vi "FTW-System-CurrentMemoryStatistics.vi"(11 "error in":errorcluster) -> (4 "DS Bytes Allocated":i64 format="%_4pbytes", 15 "error out":errorcluster)   [LabVIEW 2014]
uses:
  error/FTW-ERR-ThrowGenericError.vi
  error/FTW-ERR-ThrowError.vi
  error/FTW-ERR-CallChain.vi
  string/FTW-STR-ReplaceWhitespace.vi
panel:
  # "Inputs"
  # "Outputs"
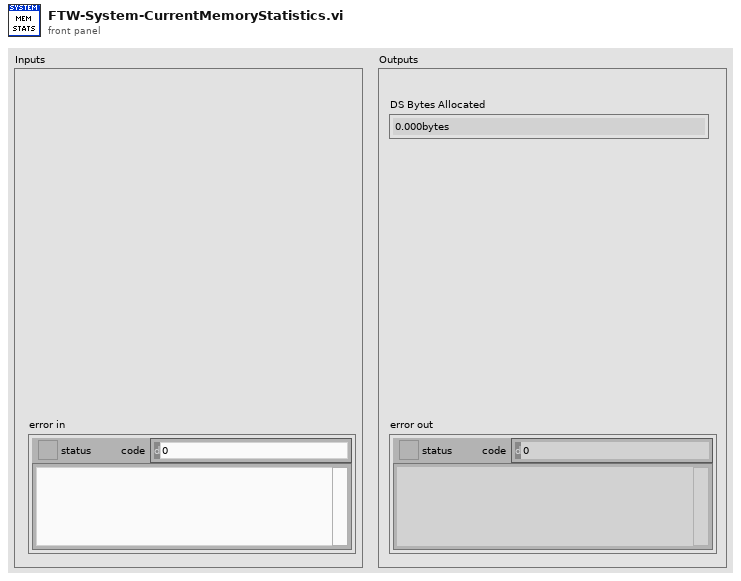
[diagram p1: front panel]
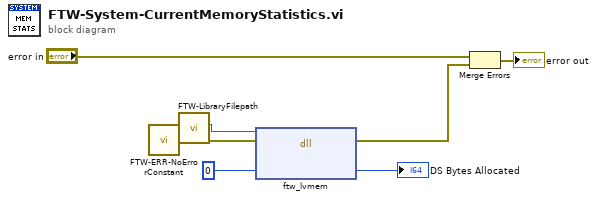
[diagram p0: block diagram]
diagram:
  n1 = call "FTW-ERR-NoErrorConstant.vi"() -> ("no error"=w4:errorcluster)
  n2 = call "FTW-LibraryFilepath.vi"("error in"=w4) -> ("error out"=w7:errorcluster, "Library Filepath"=w8:path)  [unwired: 8 in, 1 out]
  n3 = dll-call lib="?" fn="ftw_lvmem"(path in=w8, error in=w7, "Bytes Allocated"=i64 0 ("DS Max Available Handle Size")) -> (error out=w1:errorcluster, "Bytes Allocated"=→"DS Bytes Allocated":i64)  [unwired: 2 in, 1 out]
  n4 = Merge Errors("error in", w1) -> (→"error out":errorcluster)
